vi "get nano operator delay info.vi"() -> ()   [LabVIEW 2013]
panel:
  out "Files":i32
  out "File number":i32
  out "Secs delay":dbl
  out "String":string
  out "Delay Table":dbl[](array[numeric])
  out "error out":errorcluster
  in  "error in":errorcluster
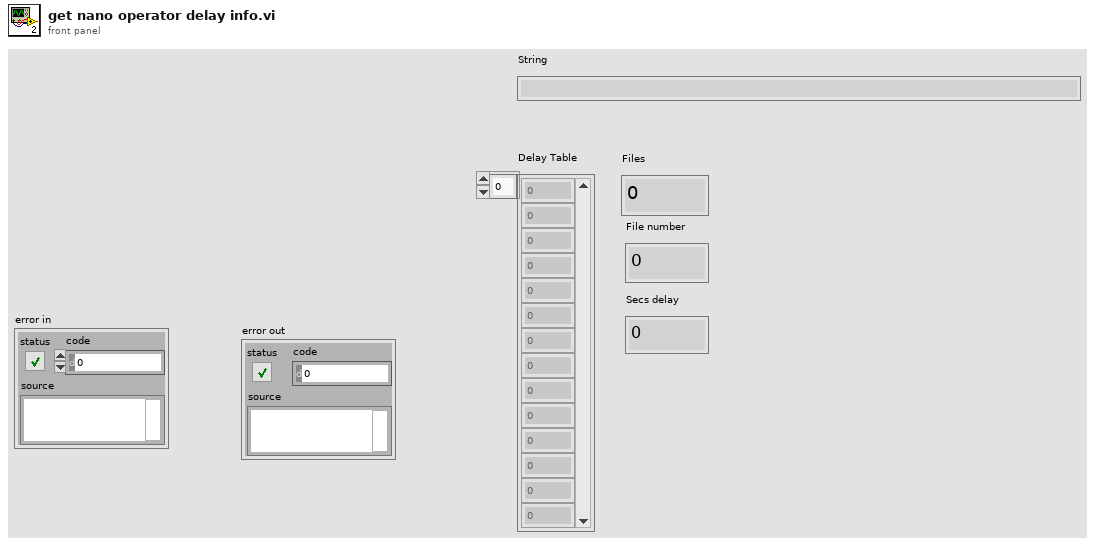
[diagram p1: front panel]
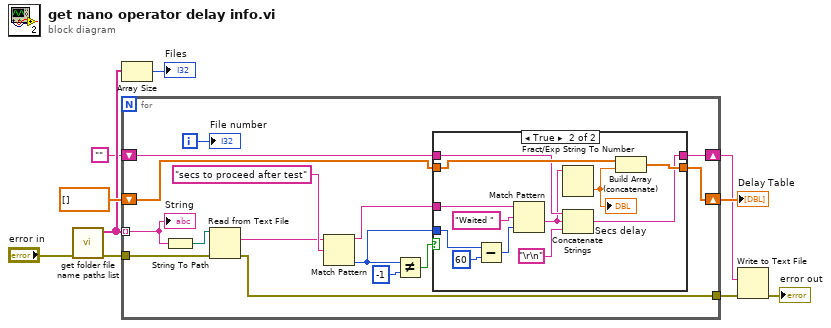
[diagram p0: block diagram]
diagram:
  n1 = call "get folder file name paths list.vi"("error in"="error in") -> ("error out"=w9:errorcluster, "File path names"=w6:string[])  [unwired: 8 in, 1 out]
  n2 = Array Size(array=w6) -> (size(s)=→"Files":i32)
  n3 = for {
    tunnel: w6 -> [w23] mode=indexing
    tunnel: w9 -> [w25]
    shift-right: [w15] -> w7
    shift-left: dbl[] [] -> [w16]
    tunnel: [w14] -> w2
    shift-right: [w11] -> w3
    shift-left: "" -> [w12]
    i -> [w13]
    n4 = String To Path(string=w23) -> (path=w24:path)
    n5 = Read from Text File(file (use dialog)=w24, error in=w25) -> (text=w21:string, error out=w14:errorcluster)  [unwired: 2 in, 2 out]
    n6 = Match Pattern(string=w21, regular expression="secs to proceed after test") -> (before substring=w18:string, offset past match=w17:i32)  [unwired: 1 in, 2 out]
    n7 = Not Equal?(x=w17, y=-1) -> (x != y?=w19:bool)
    n8 = case shown="True" w19 {
      tunnel: w18 -> [_ w36]
      tunnel: w17 -> [_ w39]
      tunnel: w16 -> [w27 w34]
      tunnel: [w27 w33] -> w15
      tunnel: w12 -> [w26 w31]
      tunnel: [w26 w29] -> w11
      frame False {
      }
      frame True {
        n9 = Subtract(x=w39, y=60) -> (x-y=w37:i32)
        n10 = Match Pattern(string=w36, regular expression="Waited ", offset (0)=w37) -> (after substring=w30:string)  [unwired: 3 out]
        n11 = Fract/Exp String To Number(string=w30) -> (number=w32:dbl)  [unwired: 3 in, 1 out]
        "Secs delay" <- w32
        n12 = Concatenate Strings(w31, w30, "\r\n") -> (w29:string)
        n13 = Build Array (concatenate)(w34, w32) -> (w33:dbl[])
      }
    }
    "String" <- w23
    "File number" <- w13
  }
  "Delay Table" <- w7
  n14 = Write to Text File(text=w3, error in=w2) -> (error out=→"error out":errorcluster)  [unwired: 2 in, 2 out]
